vi "save_log_file.vi"(11 "msg":refnum<vi>) -> ()   [LabVIEW 2016, in "MotionControl.lvlib"]
uses:
  <userlib>/MotionControl/MotionControl.lvlib
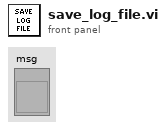
[diagram p1: front panel]
types:
  T1 = enum16{"open", "replace", "create", "open or create", "replace or create", "replace or create with confirmation"}
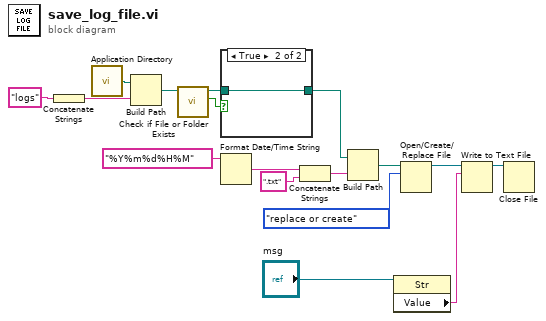
[diagram p0: block diagram]
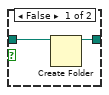
[diagram p2: hidden frame]
diagram:
  n1 = Concatenate Strings("logs") -> (w11:string)
  n2 = call <vilib>:"Application Directory.vi"() -> ("Application Directory"=w6:path)
  n3 = Build Path(base path=w6, name or relative path=w11) -> (appended path=w14:path)
  n4 = call <vilib>:"Check if File or Folder Exists.vi"("path"=w14) -> ("file or folder exists?"=w15:bool, "dup path"=w16:path)  [unwired: 8 in, 1 out]
  n5 = case shown="True" w15 {
    tunnel: w16 -> [w19 w20]
    tunnel: [w18 w20] -> w17
    frame False {
      n6 = Create Folder(path (use dialog)=w19) -> (created path=w18:path)  [unwired: 2 in, 2 out]
    }
    frame True {
    }
  }
  n7 = Format Date/Time String(time format string (%c)="%Y%m%d%H%M" ("时间格式字符串(%c)")) -> (date/time string=w3:string)  [unwired: 2 in]
  n8 = Concatenate Strings(w3, ".txt") -> (w2:string)
  n9 = Build Path(base path=w17, name or relative path=w2) -> (appended path=w5:path)
  n10 = property on="属性节点" class="Str"(reference="msg") -> ("Value"=w8:string)  [unwired: 1 in, 2 out]
  n11 = Open/Create/Replace File(file path (use dialog)=w5, operation (0:open)=T1."replace or create" ("操作(0:open)")) -> (refnum out=w9:refnum<file>)  [unwired: 4 in, 2 out]
  n12 = Write to Text File(file (use dialog)=w9, text=w8) -> (refnum out=w7:refnum<file>)  [unwired: 2 in, 2 out]
  n13 = Close File(refnum=w7) -> ()  [unwired: 1 in, 2 out]
